vi "Init.vi"(8 "error in (no error)":errorcluster, 10 "index":i32, 11 "IC_1D_Numeric":refnum<class "NI_IC_1D_Numeric.lvclass">) -> (0 "error out":errorcluster, 3 "initialized IC_1D_Numeric":refnum<class "NI_IC_1D_Numeric.lvclass">)   [LabVIEW 2020, in "NI_PDE.lvlib" / "NI_IC_1D_Numeric.lvclass"]
uses:
  <vilib>/gmath/pde.llb/ICClass/IC_1D_Numeric/NI_IC_1D_Numeric.lvclass
  <vilib>/gmath/pde.llb/ICClass/Class Type.ctl
  <vilib>/gmath/pde.llb/ICClass/IC_1D_Numeric/NI_IC_1D_Numeric.lvclass/NI_IC_1D_Numeric.ctl
  <vilib>/gmath/pde.llb/ICClass/NI_IC.lvclass
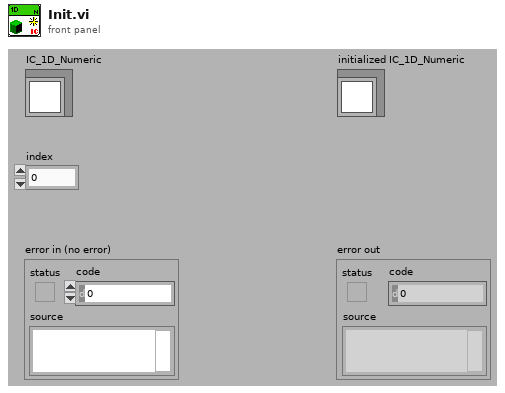
[diagram p1: front panel]
types:
  T1 = typedef "NI_PDE.lvlib/NI_IC.lvclass/Class Type.ctl" = i32
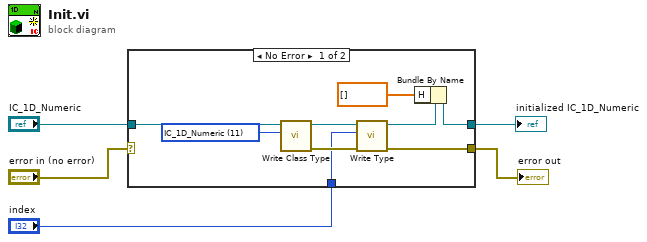
[diagram p0: block diagram]
diagram:
  n1 = case shown="No Error" "error in (no error)" {
    selector: "error in (no error)" -> [_ w15]
    tunnel: [w7 w16] -> w5
    tunnel: [w10 w15] -> w4
    tunnel: "IC_1D_Numeric" -> [w11 w16]
    tunnel: "index" -> [w6 _]
    frame No Error {
      w14 = T1 11 items=["IC"=0, "IC_1D"=10, "IC_1D_Numeric"=11, "IC_1D_VIRef"=12, "IC_2D"=20, "IC_2D_Numeric"=21, "IC_2D_VIRef"=22] ("IC class type")
      n2 = call-dynamic "Write Class Type.vi"("IC class type"=w14, "IC.lvclass in"=w11) -> ("error out"=w12:errorcluster, "IC.lvclass out"=w13:refnum<class "NI_IC_1D_Numeric.lvclass">)  [unwired: 1 in, 7 out]
      n3 = call-dynamic "Write Type.vi"("error in (no error)"=w12, "IC type"=w6, "IC.lvclass in"=w13) -> ("error out"=w10:errorcluster, "IC.lvclass out"=w8:refnum<class "NI_IC_1D_Numeric.lvclass">)  [unwired: 7 out]
      n4 = Bundle By Name(cluster=w8, "H"=dbl[] [] ("F")) -> (w7:refnum<class "NI_IC_1D_Numeric.lvclass">)
    }
    frame Error {
    }
  }
  "initialized IC_1D_Numeric" <- w5
  "error out" <- w4
